vi "OpenSession.vi"   [LabVIEW 2023]
uses:
  Open_device_2018.llb/Select_Instr.ctl
types:
  T1 = typedef "Select_Instr.ctl" = string
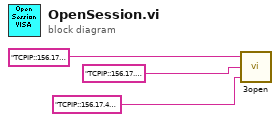
[diagram p0: block diagram]
diagram:
  n1 = call "3open.vi"("Zasilacz BM572"=T1 "TCPIP::156.17.45.35::inst18::INSTR" ("Select_Instrument"), "Komutator L201"=T1 "TCPIP::156.17.45.35::inst19::INSTR" ("Select_Instrument"), "Multimetr V553"=T1 "TCPIP::156.17.45.35::inst21::INSTR" ("Select_Instrument")) -> ()  [unwired: 1 in, 4 out]
